vi "S7Com_to_PLC(SubVI).vi"(3 "to_PLC_In":T2) -> (1 "S7Com_Data_Array_Out":T1)   [LabVIEW 2018]
doc: "Packs Labview cluster data into an array of I32 for transfer to the PLC."
uses:
  S7Com_PLC_Data.ctl
  S7Com_Data_Array.ctl
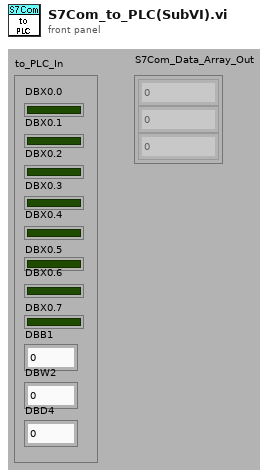
[diagram p1: front panel]
types:
  T1 = typedef "S7Com_Data_Array.ctl" = i32[]
  T2 = typedef "S7Com_PLC_Data.ctl" = cluster{"DBX0.0":bool, "DBX0.1":bool, "DBX0.2":bool, "DBX0.3":bool, "DBX0.4":bool, "DBX0.5":bool, "DBX0.6":bool, "DBX0.7":bool, "DBB1":i8, "DBW2":i16, "DBD4":i32}
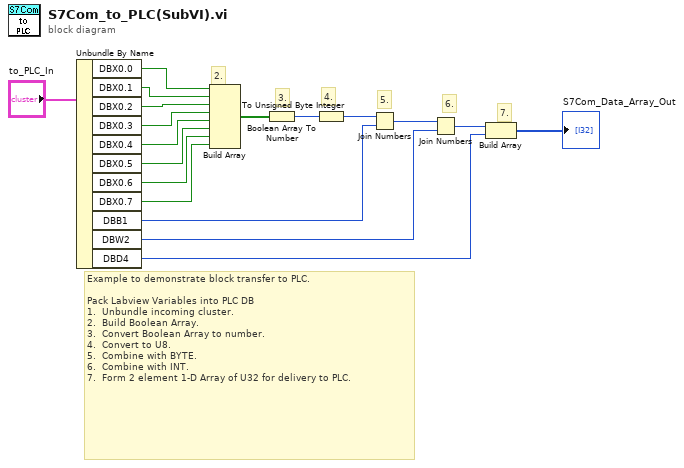
[diagram p0: block diagram]
diagram:
  # "Example to demonstrate block transfer to PLC.\n\nPack Labview Variables into PLC DB\n1.  Unbundle incoming cluster.\n2.  Build Boolean Array.\n3.  Convert Boolean Array to number.\n4.  Convert to U8.\n5.  Combine with BYTE.\n6.  Combine with INT.\n7.  Form 2 element 1-D Array of U32 for delivery to PLC."
  # "7."
  # "6."
  # "5."
  # "4."
  # "3."
  # "2."
  # "1."
  n1 = Unbundle By Name("to_PLC_In") -> ("DBX0.0"=w17:bool, "DBX0.1"=w16:bool, "DBX0.2"=w15:bool, "DBX0.3"=w14:bool, "DBX0.4"=w13:bool, "DBX0.5"=w12:bool, "DBX0.6"=w11:bool, "DBX0.7"=w10:bool, "DBB1"=w8:i8, "DBW2"=w7:i16, "DBD4"=w4:i32)
  n2 = Build Array(w17, w16, w15, w14, w13, w12, w11, w10) -> (w9:bool[])
  n3 = Boolean Array To Number(Boolean array=w9) -> (number=w2:u32)
  n4 = To Unsigned Byte Integer(number=w2) -> (unsigned 8bit integer=w1:u8)
  n5 = Join Numbers(hi=w1, lo=w8) -> ((hi.lo)=w6:u16)
  n6 = Join Numbers(hi=w6, lo=w7) -> ((hi.lo)=w5:u32)
  n7 = Build Array(w5, w4) -> (→"S7Com_Data_Array_Out":u32[])
